vi "PID_Regulering.vi"(6 "k_d":dbl, 8 "k_i":dbl, 9 "k_p":dbl, 10 "SP":dbl, 11 "DATA":dbl) -> (0 "i_pid":dbl, 1 "p_pid":dbl, 2 "e(t)":dbl, 3 "u_pid":dbl, 4 "d_pid":dbl)   [LabVIEW 2022 SP3]
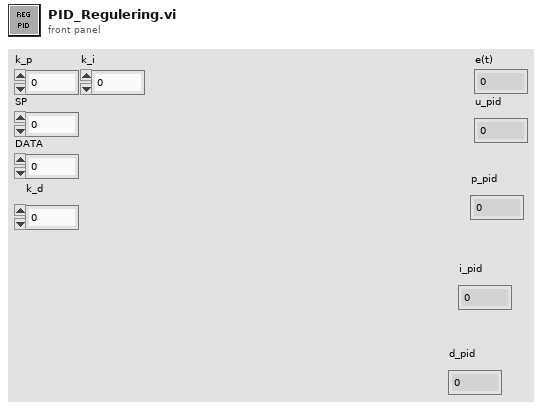
[diagram p1: front panel]
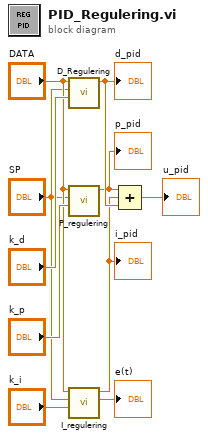
[diagram p0: block diagram]
diagram:
  n1 = call "D_Regulering.vi"("k_d"="k_d", "SP"="SP", "DATA"="DATA") -> ("u_d"=w3:dbl)  [unwired: 7 in, 1 out]
  "d_pid" <- w3
  n2 = call "P_regulering.vi"("k_p"="k_p", "SP"="SP", "DATA"="DATA") -> ("u_p"=w1:dbl)  [unwired: 6 in, 2 out]
  "p_pid" <- w1
  n3 = call "I_regulering.vi"("k_i"="k_i", "SP"="SP", "DATA"="DATA") -> ("e(t)"=→"e(t)":dbl, "u_i"=w2:dbl)  [unwired: 6 in, 1 out]
  "i_pid" <- w2
  n4 = Compound Arithmetic op=ADD(w1, w2, w3) -> (→"u_pid":dbl)
